vi "bubble.vi"(3 "Direction":bool, 4 "in":dbl[](array[numeric])) -> (0 "counter":i32, 1 "out":dbl[](array[numeric]))   [LabVIEW 2024]
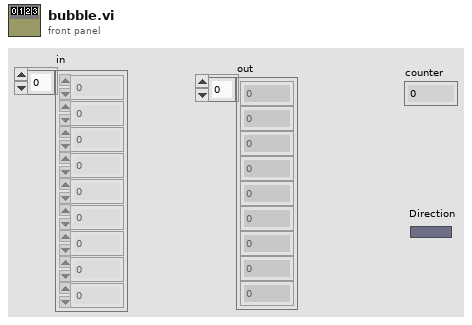
[diagram p1: front panel]
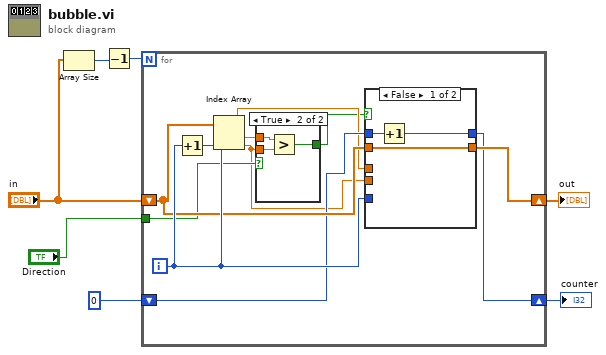
[diagram p0: block diagram]
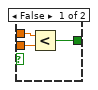
[diagram p2: hidden frame]
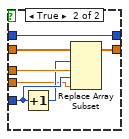
[diagram p3: hidden frame]
diagram:
  n1 = Array Size(array="in") -> (size(s)=w6:i32)
  n2 = Decrement(x=w6) -> (x-1=w5:i32)
  n3 = for {
    N: w5 -> [_]
    shift-right: [w15] -> w4
    shift-left: "in" -> [w16]
    shift-right: [w13] -> w2
    shift-left: 0 -> [w14]
    tunnel: "Direction" -> [w12]
    i -> [w17]
    n4 = Increment(x=w17) -> (x+1=w9:i32)
    n5 = Index Array(array=w16, index #1=w17, index #2=w9) -> (element #1=w11:dbl, element #2=w8:dbl)
    n6 = case shown="True" w12 {
      tunnel: w11 -> [w19 w23]
      tunnel: [w20 w22] -> w10
      tunnel: w8 -> [w18 w21]
      frame False {
        n7 = Less?(x=w19, y=w18) -> (x < y?=w20:bool)
      }
      frame True {
        n8 = Greater?(x=w23, y=w21) -> (0:w22:bool)
      }
    }
    n9 = case shown="False" w10 {
      tunnel: w17 -> [_ w31]
      tunnel: w16 -> [w26 w33]
      tunnel: w11 -> [_ w32]
      tunnel: [w26 w29] -> w15
      tunnel: w14 -> [w25 w28]
      tunnel: [w24 w28] -> w13
      tunnel: w8 -> [_ w27]
      frame False {
        n10 = Increment(x=w25) -> (x+1=w24:i32)
      }
      frame True {
        n11 = Increment(x=w31) -> (x+1=w30:i32)
        n12 = Replace Array Subset(array=w33, new element #1=w32, index #1=w30, new element #2=w27, index #2=w31) -> (w29:dbl[])
      }
    }
  }
  "out" <- w4
  "counter" <- w2
